vi "Egi1_Pitch_Roll_Yaw_Rate_Set_Get.vi"(0 "message handle in 3":u64, 1 "message handle in 2":u64, 2 "Egi1 Pitch Rate Valid":u16, 3 "Egi1 Roll Rate Valid":u16, 4 "Egi1 Roll Rate":dbl, 5 "message handle in1":u64, 6 "Egi1 Yaw Rate Valid":u16, 7 "error in (no error)":errorcluster, 8 "Egi1 Yaw Rate":dbl, 9 "Egi1 Pitch Rate":dbl) -> (14 "Egi1 Roll Rate Range Message":string, 15 "Egi1 Pitch Rate Range Message":string, 16 "Egi1 Pitch Rate Value OLD":u32 format="%.0b", 17 "Egi1 Yaw Rate Value NEW":u32 format="%08b", 20 "Egi1 Pitch Rate Value NEW":u32 format="%08b", 21 "Egi1 Roll Rate Value OLD":u32 format="%.0b", 23 "Egi1 Yaw Rate Range Message":string, 24 "Egi1 Roll Rate Value NEW":u32 format="%08b", 25 "Egi1 Yaw Rate Value OLD":u32 format="%08b", 27 "error out":errorcluster)   [LabVIEW 2023]
uses:
  <instrlib>/BTI429Lib/Private/Utility/Get BNR Data.vi
  <instrlib>/BTI429Lib/Private/Utility/Set BNR Data.vi
  <instrlib>/BTI429Lib/BTI429LV.lvlib
  <instrlib>/BTI429Lib/Private/Utility/Set BNR SSM.vi
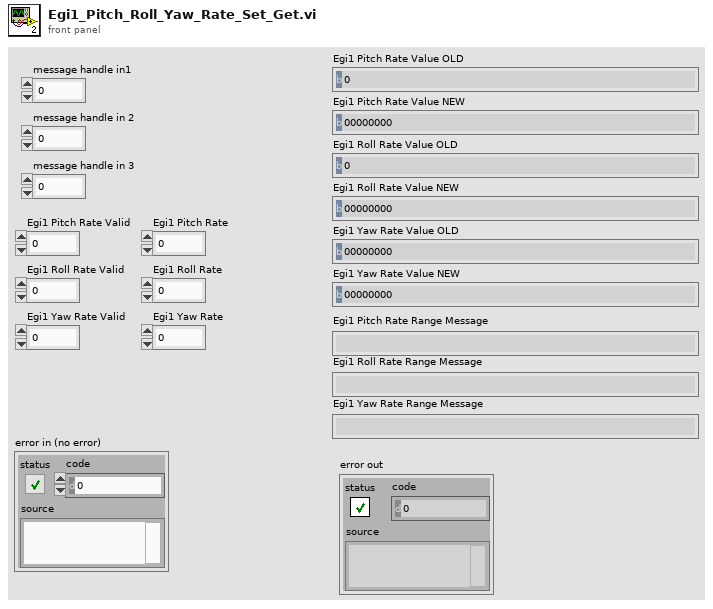
[diagram p1: front panel]
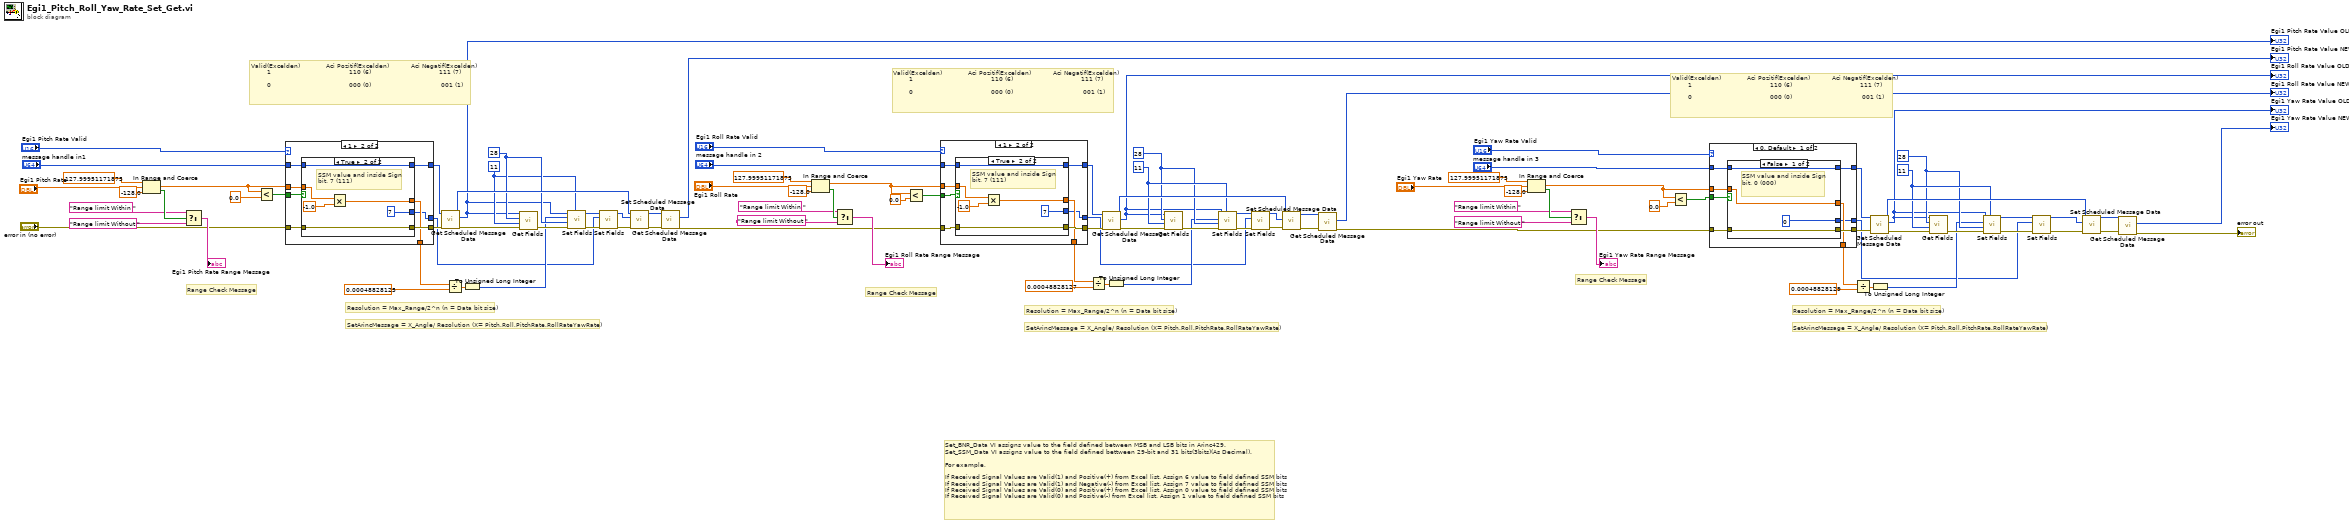
[diagram p0: block diagram]
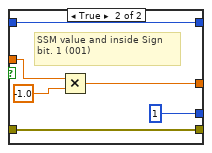
[diagram p2: hidden frame]
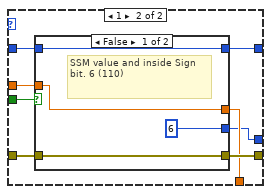
[diagram p3: hidden frame]
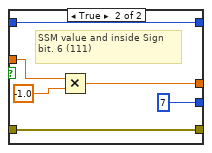
[diagram p4: hidden frame]
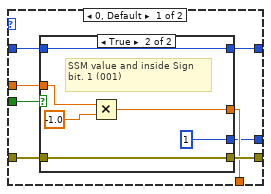
[diagram p5: hidden frame]
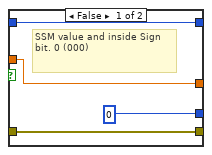
[diagram p6: hidden frame]
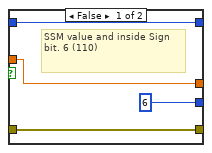
[diagram p7: hidden frame]
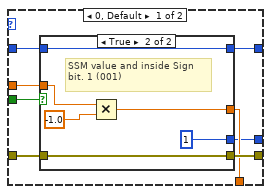
[diagram p8: hidden frame]
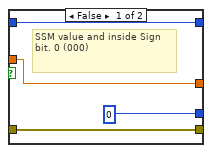
[diagram p9: hidden frame]
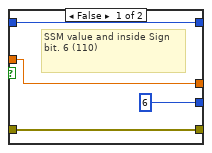
[diagram p10: hidden frame]
diagram:
  w95 = u16 28 ("most significant bit")
  w96 = u16 11 ("least significant bit")
  w74 = u16 28 ("most significant bit")
  w75 = u16 11 ("least significant bit")
  w83 = u16 28 ("most significant bit")
  w82 = u16 11 ("least significant bit")
  # "Range Check Message"
  # "SetArincMessage = X_Angle/ Resolution (X= Pitch,Roll,PitchRate,RollRateYawRate)"
  # "Resolution = Max_Range/2^n (n = Data bit size)"
  # "Range Check Message"
  # "Range Check Message"
  # "SetArincMessage = X_Angle/ Resolution (X= Pitch,Roll,PitchRate,RollRateYawRate)"
  # "Resolution = Max_Range/2^n (n = Data bit size)"
  # "SetArincMessage = X_Angle/ Resolution (X= Pitch,Roll,PitchRate,RollRateYawRate)"
  # "Resolution = Max_Range/2^n (n = Data bit size)"
  # "Set_BNR_Data VI assigns value to the field defined between MSB and LSB bits in Arinc429.\nSet_SSM_Data VI assigns value to the field defined bettween 29-bit and 31 bits(3bits)(As Decimal).\n\nFor example,\n\nIf Received Signal Values are Valid(1) and Positive(+) from Excel list. Assign 6 value to field defined SSM bits\nIf Received Signal Values are Valid(1) and Negative(-) from Excel list. Assign 7 value to field defined SSM bits\nIf Received Signal Values are Valid(0) and Positive(+) from Excel list. Assign 0 value to field defined SSM bits\nIf Received Signal Values are Valid(0) and Positive(-) from Excel list. Assign 1 value to field defined SSM bits"
  # "Valid(Excelden)             Aci Pozitif(Excelden)           Aci Negatif(Excelden) \n        1                                       110 (6)                                  111 (7)\n\n        0                                       000 (0)                                   001 (1)"
  # "Valid(Excelden)             Aci Pozitif(Excelden)           Aci Negatif(Excelden) \n        1                                       110 (6)                                  111 (7)\n\n        0                                       000 (0)                                   001 (1)"
  # "Valid(Excelden)             Aci Pozitif(Excelden)           Aci Negatif(Excelden) \n        1                                       110 (6)                                  111 (7)\n\n        0                                       000 (0)                                   001 (1)"
  n1 = In Range and Coerce(upper limit=127.99951171875, x="Egi1 Pitch Rate", lower limit=-128.0) -> (coerced(x)=w35:dbl, In Range?=w59:bool)
  n2 = Select(t="Range limit Within ", s=w59, f="Range limit Without ") -> (s? t:f=→"Egi1 Pitch Rate Range Message":string)
  n3 = Less?(x=w35, y=0.0) -> (x < y?=w34:bool)
  n4 = case shown="1" "Egi1 Pitch Rate Valid" {
    tunnel: [w107 w126] -> w33
    tunnel: [w105 w125] -> w38
    tunnel: "error in (no error)" -> [w108 w124]
    tunnel: "message handle in1" -> [w106 w123]
    tunnel: w34 -> [w101 w122]
    tunnel: [w103 w121] -> w36
    tunnel: w35 -> [w104 w120]
    tunnel: [w102 w119] -> w28
    frame 0, Default {
      n5 = case shown="True" w101 {
        tunnel: w104 -> [w112 w114]
        tunnel: [w112 w117] -> w103
        tunnel: w106 -> [w111 w116]
        tunnel: w108 -> [w110 w115]
        tunnel: [w111 w116] -> w105
        tunnel: [w110 w115] -> w107
        tunnel: [u16 0 ("value") u16 1 ("value")] -> w102
        frame False {
          # "SSM value and inside Sign bit. 0 (000)"
        }
        frame True {
          # "SSM value and inside Sign bit. 1 (001)"
          n6 = Multiply(x=w114, y=-1.0) -> (x*y=w117:dbl)
        }
      }
    }
    frame 1 {
      n7 = case shown="True" w122 {
        tunnel: w120 -> [w130 w135]
        tunnel: [w130 w134] -> w121
        tunnel: w123 -> [w129 w133]
        tunnel: w124 -> [w128 w132]
        tunnel: [w129 w133] -> w125
        tunnel: [w128 w132] -> w126
        tunnel: [u16 6 ("value") u16 7 ("value")] -> w119
        frame False {
          # "SSM value and inside Sign bit. 6 (110)"
        }
        frame True {
          # "SSM value and inside Sign bit. 7 (111)"
          n8 = Multiply(x=w135, y=-1.0) -> (x*y=w134:dbl)
        }
      }
    }
  }
  n9 = call <instrlib>:"Get Scheduled Message Data.vi"("error in (no error)"=w33, "message handle in"=w38) -> ("error out"=w86:errorcluster, "value"=w68:u32, "message handle out"=w84:u64)  [unwired: 7 in]
  "Egi1 Pitch Rate Value OLD" <- w68
  n10 = Divide(x=w36, y=0.00048828125) -> (x/y=w79:dbl)
  n11 = To Unsigned Long Integer(number=w79) -> (unsigned 32bit integer=w73:u32)
  n12 = call-poly <instrlib>:"Get Fields.vi"("error in (no error)"=w86, "least significant bit"=w82, "most significant bit"=w83, "message"=w68) -> ("error out"=w85:errorcluster)  [unwired: 6 in, 1 out]
  n13 = call-poly <instrlib>:"Set Fields.vi"("least significant bit"=w82, "error in (no error)"=w85, "most significant bit"=w83, "value"=w73, "message"=w68) -> ("error out"=w32:errorcluster, "message out"=w29:u32)  [unwired: 5 in]
  n14 = call-poly <instrlib>:"Set Fields.vi"("error in (no error)"=w32, "value"=w28, "message"=w29) -> ("error out"=w31:errorcluster, "message out"=w30:u32)  [unwired: 7 in]
  n15 = call <instrlib>:"Set Scheduled Message Data.vi"("error in (no error)"=w31, "value"=w30, "message handle in"=w84) -> ("error out"=w63:errorcluster, "message handle out"=w62:u64)  [unwired: 7 in]
  n16 = call <instrlib>:"Get Scheduled Message Data.vi"("error in (no error)"=w63, "message handle in"=w62) -> ("error out"=w24:errorcluster, "value"=→"Egi1 Pitch Rate Value NEW":u32)  [unwired: 7 in, 1 out]
  n17 = In Range and Coerce(upper limit=127.99951171875, x="Egi1 Roll Rate", lower limit=-128.0) -> (coerced(x)=w26:dbl, In Range?=w52:bool)
  n18 = Select(t="Range limit Within ", s=w52, f="Range limit Without ") -> (s? t:f=→"Egi1 Roll Rate Range Message":string)
  n19 = Less?(x=w26, y=0.0) -> (x < y?=w25:bool)
  n20 = case shown="1" "Egi1 Roll Rate Valid" {
    tunnel: [w143 w162] -> w22
    tunnel: [w139 w161] -> w21
    tunnel: w24 -> [w144 w160]
    tunnel: "message handle in 2" -> [w138 w159]
    tunnel: w25 -> [w137 w158]
    tunnel: [w141 w157] -> w23
    tunnel: w26 -> [w142 w156]
    tunnel: [w140 w155] -> w16
    frame 0, Default {
      n21 = case shown="True" w137 {
        tunnel: w142 -> [w148 w150]
        tunnel: [w148 w153] -> w141
        tunnel: w138 -> [w147 w152]
        tunnel: w144 -> [w146 w151]
        tunnel: [w147 w152] -> w139
        tunnel: [w146 w151] -> w143
        tunnel: [u16 0 ("value") u16 1 ("value")] -> w140
        frame False {
          # "SSM value and inside Sign bit. 0 (000)"
        }
        frame True {
          # "SSM value and inside Sign bit. 1 (001)"
          n22 = Multiply(x=w150, y=-1.0) -> (x*y=w153:dbl)
        }
      }
    }
    frame 1 {
      n23 = case shown="True" w158 {
        tunnel: w156 -> [w166 w171]
        tunnel: [w166 w170] -> w157
        tunnel: w159 -> [w165 w169]
        tunnel: w160 -> [w164 w168]
        tunnel: [w165 w169] -> w161
        tunnel: [w164 w168] -> w162
        tunnel: [u16 6 ("value") u16 7 ("value")] -> w155
        frame False {
          # "SSM value and inside Sign bit. 6 (110)"
        }
        frame True {
          # "SSM value and inside Sign bit. 7 (111)"
          n24 = Multiply(x=w171, y=-1.0) -> (x*y=w170:dbl)
        }
      }
    }
  }
  n25 = Divide(x=w23, y=0.00048828127) -> (x/y=w70:dbl)
  n26 = call <instrlib>:"Get Scheduled Message Data.vi"("error in (no error)"=w22, "message handle in"=w21) -> ("error out"=w77:errorcluster, "value"=w67:u32, "message handle out"=w78:u64)  [unwired: 7 in]
  "Egi1 Roll Rate Value OLD" <- w67
  n27 = To Unsigned Long Integer(number=w70) -> (unsigned 32bit integer=w69:u32)
  n28 = call-poly <instrlib>:"Get Fields.vi"("error in (no error)"=w77, "least significant bit"=w75, "most significant bit"=w74, "message"=w67) -> ("error out"=w76:errorcluster)  [unwired: 6 in, 1 out]
  n29 = call-poly <instrlib>:"Set Fields.vi"("least significant bit"=w75, "error in (no error)"=w76, "most significant bit"=w74, "value"=w69, "message"=w67) -> ("error out"=w20:errorcluster, "message out"=w17:u32)  [unwired: 5 in]
  n30 = call-poly <instrlib>:"Set Fields.vi"("error in (no error)"=w20, "value"=w16, "message"=w17) -> ("error out"=w19:errorcluster, "message out"=w18:u32)  [unwired: 7 in]
  n31 = call <instrlib>:"Set Scheduled Message Data.vi"("error in (no error)"=w19, "value"=w18, "message handle in"=w78) -> ("error out"=w66:errorcluster, "message handle out"=w65:u64)  [unwired: 7 in]
  n32 = call <instrlib>:"Get Scheduled Message Data.vi"("error in (no error)"=w66, "message handle in"=w65) -> ("error out"=w15:errorcluster, "value"=→"Egi1 Roll Rate Value NEW":u32)  [unwired: 7 in, 1 out]
  n33 = In Range and Coerce(upper limit=127.99951171875, x="Egi1 Yaw Rate", lower limit=-128.0) -> (coerced(x)=w13:dbl, In Range?=w45:bool)
  n34 = Select(t="Range limit Within ", s=w45, f="Range limit Without ") -> (s? t:f=→"Egi1 Yaw Rate Range Message":string)
  n35 = Less?(x=w13, y=0.0) -> (x < y?=w14:bool)
  n36 = case shown="0, Default" "Egi1 Yaw Rate Valid" {
    tunnel: [w179 w198] -> w10
    tunnel: [w175 w197] -> w11
    tunnel: w15 -> [w180 w196]
    tunnel: "message handle in 3" -> [w174 w195]
    tunnel: w14 -> [w173 w194]
    tunnel: [w177 w193] -> w9
    tunnel: w13 -> [w178 w192]
    tunnel: [w176 w191] -> w4
    frame 0, Default {
      n37 = case shown="False" w173 {
        tunnel: w178 -> [w184 w186]
        tunnel: [w184 w189] -> w177
        tunnel: w174 -> [w183 w188]
        tunnel: w180 -> [w182 w187]
        tunnel: [w183 w188] -> w175
        tunnel: [w182 w187] -> w179
        tunnel: [u16 0 ("value") u16 1 ("value")] -> w176
        frame False {
          # "SSM value and inside Sign bit. 0 (000)"
        }
        frame True {
          # "SSM value and inside Sign bit. 1 (001)"
          n38 = Multiply(x=w186, y=-1.0) -> (x*y=w189:dbl)
        }
      }
    }
    frame 1 {
      n39 = case shown="False" w194 {
        tunnel: w192 -> [w202 w207]
        tunnel: [w202 w206] -> w193
        tunnel: w195 -> [w201 w205]
        tunnel: w196 -> [w200 w204]
        tunnel: [w201 w205] -> w197
        tunnel: [w200 w204] -> w198
        tunnel: [u16 6 ("value") u16 7 ("value")] -> w191
        frame False {
          # "SSM value and inside Sign bit. 6 (110)"
        }
        frame True {
          # "SSM value and inside Sign bit. 6 (111)"
          n40 = Multiply(x=w207, y=-1.0) -> (x*y=w206:dbl)
        }
      }
    }
  }
  n41 = Divide(x=w9, y=0.00048828129) -> (x/y=w92:dbl)
  n42 = call <instrlib>:"Get Scheduled Message Data.vi"("error in (no error)"=w10, "message handle in"=w11) -> ("error out"=w98:errorcluster, "value"=w90:u32, "message handle out"=w99:u64)  [unwired: 7 in]
  "Egi1 Yaw Rate Value OLD" <- w90
  n43 = To Unsigned Long Integer(number=w92) -> (unsigned 32bit integer=w91:u32)
  n44 = call-poly <instrlib>:"Get Fields.vi"("error in (no error)"=w98, "least significant bit"=w96, "most significant bit"=w95, "message"=w90) -> ("error out"=w97:errorcluster)  [unwired: 6 in, 1 out]
  n45 = call-poly <instrlib>:"Set Fields.vi"("least significant bit"=w96, "error in (no error)"=w97, "most significant bit"=w95, "value"=w91, "message"=w90) -> ("error out"=w8:errorcluster, "message out"=w5:u32)  [unwired: 5 in]
  n46 = call-poly <instrlib>:"Set Fields.vi"("error in (no error)"=w8, "value"=w4, "message"=w5) -> ("error out"=w7:errorcluster, "message out"=w6:u32)  [unwired: 7 in]
  n47 = call <instrlib>:"Set Scheduled Message Data.vi"("error in (no error)"=w7, "value"=w6, "message handle in"=w99) -> ("error out"=w89:errorcluster, "message handle out"=w88:u64)  [unwired: 7 in]
  n48 = call <instrlib>:"Get Scheduled Message Data.vi"("error in (no error)"=w89, "message handle in"=w88) -> ("error out"=→"error out":errorcluster, "value"=→"Egi1 Yaw Rate Value NEW":u32)  [unwired: 7 in, 1 out]
